vi "measurementChanged.vi"(8 "error in (no error)":errorcluster, 11 "WeatherData.lvclass":refnum<class "WeatherData.lvclass">) -> (0 "error out":errorcluster, 3 "WeatherData.lvclass 2":refnum<class "WeatherData.lvclass">)   [LabVIEW 2020, in "WeatherData.lvclass"]
uses:
  WeatherData.lvclass
  WeatherData.lvclass/WeatherData.ctl
panel:
  # "Connector Pane"
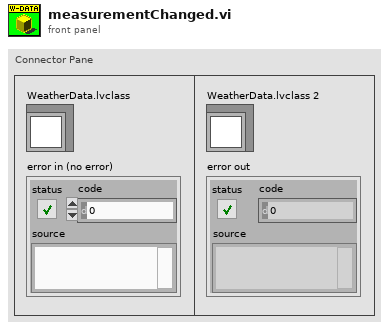
[diagram p1: front panel]
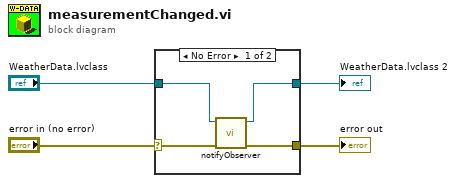
[diagram p0: block diagram]
diagram:
  n1 = case shown="No Error" "error in (no error)" {
    selector: "error in (no error)" -> [w7 w10]
    tunnel: "WeatherData.lvclass" -> [w8 w9]
    tunnel: [w6 w9] -> w2
    tunnel: [w5 w10] -> w1
    frame No Error {
      n2 = call-dynamic "notifyObserver.vi"("error in (no error)"=w7, "WeatherData.lvclass"=w8) -> ("error out"=w5:errorcluster, "WeatherData.lvclass 2"=w6:refnum<class "WeatherData.lvclass">)  [unwired: 8 in]
    }
    frame Error {
    }
  }
  "error out" <- w1
  "WeatherData.lvclass 2" <- w2
